vi "Set_First_AI_Task_name.vi"(8 "error in (no error)":errorcluster, 10 "Name":string, 11 "DAQmxTaksContainer_General in":refnum<class "DAQmxTaksContainer_General.lvclass">) -> (0 "error out":errorcluster, 3 "DAQmxTaksContainer_General out":refnum<class "DAQmxTaksContainer_General.lvclass">)   [LabVIEW 2020, in "DAQmxTaksContainer_General.lvclass"]
uses:
  DAQmxTaksContainer_General.lvclass
  DAQmxTaksContainer_General.lvclass/DAQmxTaksContainer_General.ctl
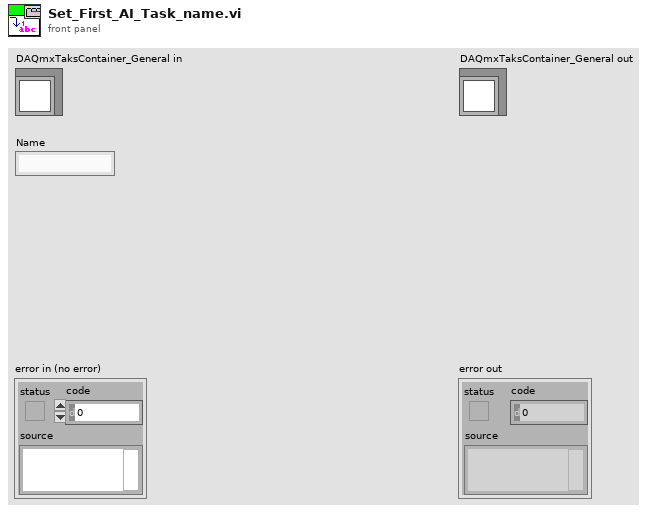
[diagram p1: front panel]
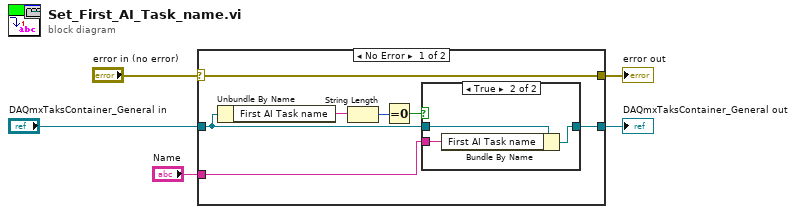
[diagram p0: block diagram]
diagram:
  n1 = case shown="No Error" "error in (no error)" {
    selector: "error in (no error)" -> [w12 w18]
    tunnel: [w12 w18] -> w4
    tunnel: [w6 w17] -> w2
    tunnel: "DAQmxTaksContainer_General in" -> [w7 w17]
    tunnel: "Name" -> [w8 _]
    frame No Error {
      n2 = Unbundle By Name(w7) -> ("First AI Task name"=w11:string)
      n3 = String Length(string=w11) -> (length=w10:i32)
      n4 = Equal To 0?(x=w10) -> (x = 0?=w9:bool)
      n5 = case shown="True" w9 {
        tunnel: w8 -> [_ w14]
        tunnel: w7 -> [w13 w16]
        tunnel: [w13 w15] -> w6
        frame False {
        }
        frame True {
          n6 = Bundle By Name(cluster=w16, "First AI Task name"=w14) -> (w15:refnum<class "DAQmxTaksContainer_General.lvclass">)
        }
      }
    }
    frame Error {
    }
  }
  "error out" <- w4
  "DAQmxTaksContainer_General out" <- w2
